vi "DolzinaVektorja.vi"(9 "z":dbl, 10 "y":dbl, 11 "x":dbl) -> (3 "magnitude":dbl)   [LabVIEW 2021]
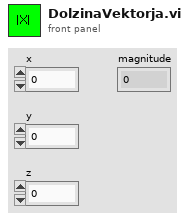
[diagram p1: front panel]
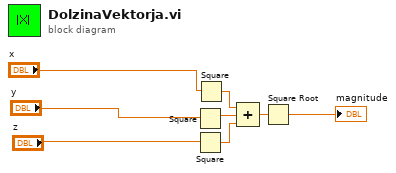
[diagram p0: block diagram]
diagram:
  n1 = Square(x="y") -> (x^2=w3:dbl)
  n2 = Square(x="z") -> (x^2=w2:dbl)
  n3 = Square(x="x") -> (x^2=w4:dbl)
  n4 = Compound Arithmetic op=ADD(w4, w3, w2) -> (w1:dbl)
  n5 = Square Root(x=w1) -> (sqrt(x)=→"magnitude":dbl)
